vi "test.vi"() -> ()   [LabVIEW 2010]
uses:
  ROS/Code/SubVIs/_ROSDirection.ctl
  ROS/Code/_ROSDefinition.vi
  ROS/Code/Console/Servers/ServerSubs/TopicDef.ctl
  ROS/parsing/std_msgs/subs/parse_time_scalar.vi
  ROS/parsing/std_msgs/subs/parse_u8_scalar.vi
  ROS/parsing/std_msgs/subs/parse_string_array.vi
panel:
  out "strings":string[](array[string])
  out "WorldProperties":T1
  out "Time":cluster{"secs":i32, "nsecs":i32}
  in  "Twist":T2
  in  "Pose":T3 {"Point"."x" scale=-3.0..3.0}
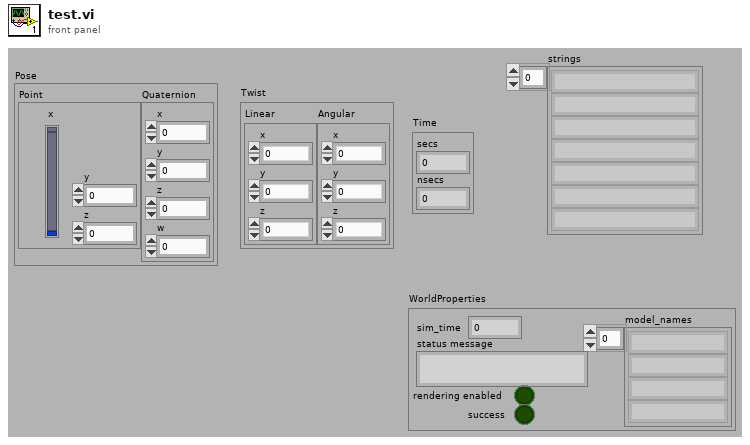
[diagram p1: front panel]
types:
  T1 = cluster{"sim_time":dbl, "model_names":string[], "rendering enabled":bool, "success":bool, "status message":string}
  T2 = cluster{"Linear":cluster{"x":dbl, "y":dbl, "z":dbl}, "Angular":cluster{"x":dbl, "y":dbl, "z":dbl}}
  T3 = cluster{"Point":cluster{"x":dbl, "y":dbl, "z":dbl}, "Quaternion":cluster{"x":dbl, "y":dbl, "z":dbl, "w":dbl}}
  T4 = enum16{"GazeboPub", "GazeboSub", "BaxterPub", "GazeboService", "BaxterService"}
  T5 = typedef "TopicDef.ctl" = cluster{"Topic":string, "Type":string, "Action":T6, "Update (ms)":u16, "write queue":u16}
  T6 = typedef "_ROSDirection.ctl" = enum16{"Node", "Publisher", "Subscriber", "Service Client"}
  T7 = typedef "_ROSControl.ctl" = cluster{"topic port":u16, "Node":string, "topic":string, "type":string, "node port":u32, "error ":errorcluster, "Direction":T6, "APIs":string[], "Update (ms)":u16, "write queue":u16}
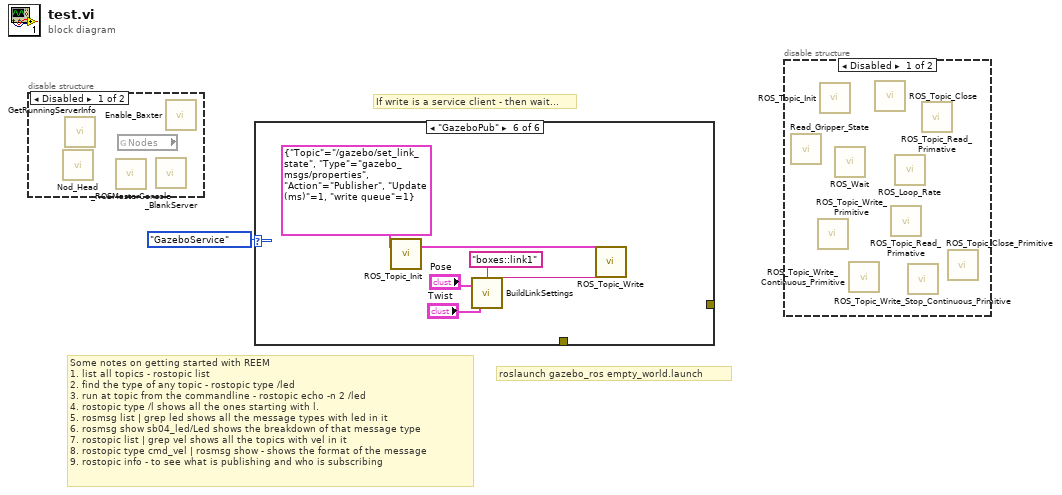
[diagram p0: block diagram]
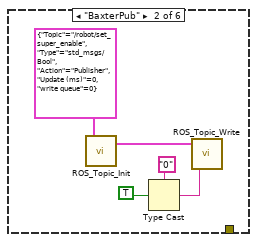
[diagram p3: hidden frame]
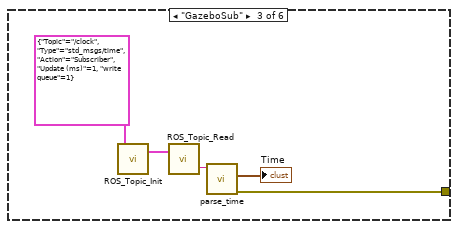
[diagram p4: hidden frame]
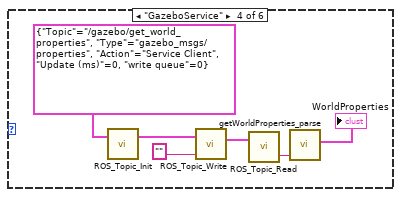
[diagram p5: hidden frame]
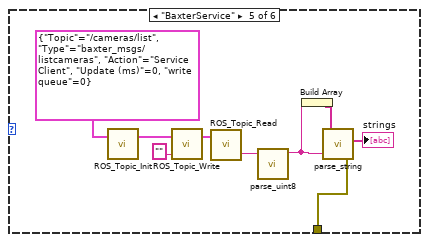
[diagram p6: hidden frame]
diagram:
  # "roslaunch gazebo_ros empty_world.launch"
  # "Some notes on getting started with REEM\n1. list all topics - rostopic list\n2. find the type of any topic - rostopic type /led\n3. run at topic from the commandline - rostopic echo -n 2 /led\n4. rostopic type /l shows all the ones starting with l.\n5. rosmsg list | grep led shows all the message types with led in it\n6. rosmsg show sb04_led/Led shows the breakdown of that message type\n7. rostopic list | grep vel shows all the topics with vel in it\n8. rostopic type cmd_vel | rosmsg show - shows the format of the message\n9. rostopic info - to see what is publishing and who is subscribing"
  # "If write is a service client - then wait..."
  n1 = disable-structure shown="Disabled" {
    frame Disabled {
      n2 = call "Nod_Head.vi"() -> ()  [unwired: 4 in, 1 out]
      n3 = call "GetRunningServerInfo.vi"() -> ()  [unwired: 2 in, 3 out]
      n4 = call "_ROSMasterConsole.vi"() -> ()  [unwired: 12 in]
      n5 = global read "_ROSDefinition.vi" "Nodes"() -> ()  [unwired: 1 out]
      n6 = call "_BlankServer.vi"() -> ()  [unwired: 4 in]
      n7 = call "Enable_Baxter.vi"() -> ()  [unwired: 4 in, 1 out]
    }
    frame Enabled {
    }
  }
  n8 = case shown="\"GazeboPub\"" T4."GazeboService" {
    tunnel: [_ _ _ _ w22 _] -> _
    tunnel: [_ _ w7 _ _ _] -> _
    frame Default {
    }
    frame "BaxterPub" {
      n9 = call "ROS_Topic_Init.vi"("Definitions"=T5 {"Topic"="/robot/set_super_enable", "Type"="std_msgs/Bool", "Action"=enum."Publisher", "Update (ms)"=0, "write queue"=0}) -> ("ROS out"=w5:T7)  [unwired: 2 in]
      n10 = Type Cast(type="0" ("Msg in"), x=TRUE) -> (*(type *) &x=w2:string)
      n11 = call "ROS_Topic_Write.vi"("Msg in"=w2, "ROS in"=w5) -> ()  [unwired: 2 in, 1 out]
    }
    frame "GazeboSub" {
      n12 = call "ROS_Topic_Init.vi"("Definitions"=T5 {"Topic"="/clock", "Type"="std_msgs/time", "Action"=enum."Subscriber", "Update (ms)"=1, "write queue"=1}) -> ("ROS out"=w8:T7)  [unwired: 2 in]
      n13 = call "ROS_Topic_Read.vi"("ROS in"=w8) -> ("Reply"=w10:string)  [unwired: 1 in, 1 out]
      n14 = call-poly "parse_time.vi"("msg in"=w10) -> ("error out"=w7:errorcluster, "Time"=→"Time":cluster{"secs":i32, "nsecs":i32})  [unwired: 4 in, 1 out]
    }
    frame "GazeboService" {
      n15 = call "ROS_Topic_Init.vi"("Definitions"=T5 {"Topic"="/gazebo/get_world_properties", "Type"="gazebo_msgs/properties", "Action"=enum."Service Client", "Update (ms)"=0, "write queue"=0}) -> ("ROS out"=w17:T7)  [unwired: 2 in]
      n16 = call "ROS_Topic_Write.vi"("Msg in"="", "ROS in"=w17) -> ("ROS out"=w13:T7)  [unwired: 2 in]
      n17 = call "ROS_Topic_Read.vi"("ROS in"=w13) -> ("Reply"=w12:string)  [unwired: 1 in, 1 out]
      n18 = call "getWorldProperties_parse.vi"("msg in"=w12) -> ("WorldProperties"=→"WorldProperties":T1)  [unwired: 8 in, 2 out]
    }
    frame "BaxterService" {
      n19 = call "ROS_Topic_Init.vi"("Definitions"=T5 {"Topic"="/cameras/list", "Type"="baxter_msgs/listcameras", "Action"=enum."Service Client", "Update (ms)"=0, "write queue"=0}) -> ("ROS out"=w26:T7)  [unwired: 2 in]
      n20 = call "ROS_Topic_Write.vi"("Msg in"="", "ROS in"=w26) -> ("ROS out"=w24:T7)  [unwired: 2 in]
      n21 = call "ROS_Topic_Read.vi"("ROS in"=w24) -> ("Reply"=w19:string)  [unwired: 1 in, 1 out]
      n22 = call-poly "parse_uint8.vi"("msg in"=w19) -> ("msg out"=w18:string)  [unwired: 4 in, 2 out]
      n23 = Build Array(w18) -> (w21:string[])
      n24 = call-poly "parse_string.vi"("type"=w21, "msg in"=w18) -> ("error out"=w22:errorcluster, "strings"=→"strings":string[])  [unwired: 3 in, 1 out]
    }
    frame "GazeboPub" {
      n25 = call "ROS_Topic_Init.vi"("Definitions"=T5 {"Topic"="/gazebo/set_link_state", "Type"="gazebo_msgs/properties", "Action"=enum."Publisher", "Update (ms)"=1, "write queue"=1}) -> ("ROS out"=w28:T7)  [unwired: 2 in]
      n26 = call "BuildLinkSettings.vi"("Twist"="Twist", "Pose"="Pose", "link to move"="boxes::link1") -> ("msg out"=w32:string)  [unwired: 1 in]
      n27 = call "ROS_Topic_Write.vi"("Msg in"=w32, "ROS in"=w28) -> ()  [unwired: 2 in, 1 out]
    }
  }
  n28 = disable-structure shown="Disabled" {
    frame Disabled {
      n29 = call "Read_Gripper_State.vi"() -> ()  [unwired: 3 in, 2 out]
      n30 = call "ROS_Topic_Write_Primitive.vi"() -> ()  [unwired: 3 in, 1 out]
      n31 = call "ROS_Topic_Init.vi"() -> ()  [unwired: 3 in, 1 out]
      n32 = call "ROS_Wait.vi"() -> ()  [unwired: 6 in, 1 out]
      n33 = call "ROS_Topic_Write_Continuous_Primitive.vi"() -> ()  [unwired: 3 in, 1 out]
      n34 = call "ROS_Topic_Close.vi"() -> ()  [unwired: 4 in, 1 out]
      n35 = call "ROS_Topic_Read_Primative.vi"() -> ()  [unwired: 2 in, 2 out]
      n36 = call "ROS_Loop_Rate.vi"() -> ()  [unwired: 5 in, 2 out]
      n37 = call "ROS_Topic_Write_Stop_Continuous_Primitive.vi"() -> ()  [unwired: 3 in, 1 out]
      n38 = call "ROS_Topic_Read_Primative.vi"() -> ()  [unwired: 2 in, 2 out]
      n39 = call "ROS_Topic_Close_Primitive.vi"() -> ()  [unwired: 3 in, 1 out]
    }
    frame Enabled {
    }
  }
